vi "Input Selector.vi"(2 "elements":u32[](array[numeric]), 3 "input points":dbl[](array[numeric]) format="%.2f") -> (1 "output points":dbl[](array[numeric]) format="%.2f")   [LabVIEW 2020, in "NI_AdvCtrl_nonlinear.lvlib"]
doc: "LabVIEW no longer supports this VI. You can obtain similar functionality by installing the LabVIEW Simulation Module.\n\nCollects some specific channels from a given list of channels."
uses:
  <vilib>/addons/control/advanced/NI_AdvCtrl_nonlinear.lvlib
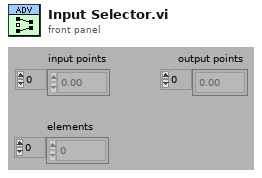
[diagram p1: front panel]
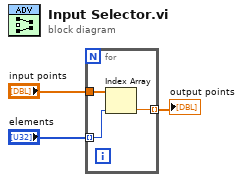
[diagram p0: block diagram]
diagram:
  n1 = for {
    tunnel: "input points" -> [w6]
    tunnel: "elements" -> [w5] mode=indexing
    tunnel: [w4] -> w1 mode=indexing
    n2 = Index Array(array=w6, index=w5) -> (element=w4:dbl)
  }
  "output points" <- w1
